vi "Playground.vi"() -> ()   [LabVIEW 2020]
uses:
  Maui 2.0/Maui 2.0.lvclass
  C:/Program Files (x86)/National Instruments/LabVIEW 2020/vi.lib/JKI/JKI SMO/SMO/SMO.lvclass
  <vilib>/JKI/JKI SMO/SMO/SMO.lvclass
panel:
  in  "Stop":bool
  in  "Ring 2":u16(ring) items=["Maui 2.0", "None"]
  in  "Ring":u16(ring) items=["Maui 2.0", "None"]
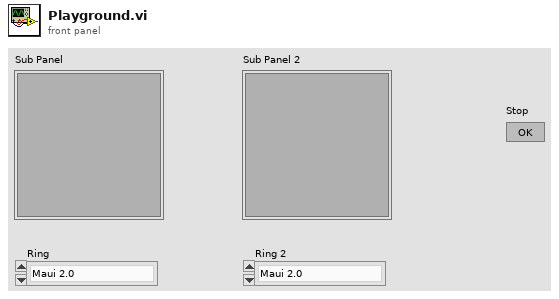
[diagram p1: front panel]
types:
  T1 = cluster{"Ring":refnum<vi>, "Sub Panel":refnum<vi>}
  T2 = cluster{"Ring 2":refnum<vi>, "Sub Panel 2":refnum<vi>}
  T3 = cluster{"Ring 2":refnum<vi>, "Sub Panel 2":refnum<vi>}[]
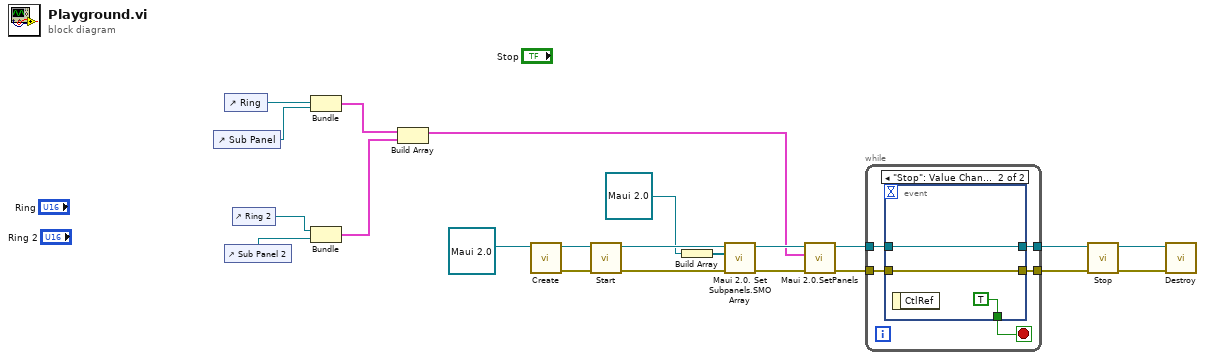
[diagram p0: block diagram]
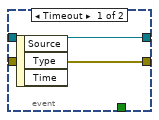
[diagram p2: hidden frame]
diagram:
  n1 = control-ref of="Sub Panel"() -> (w21:refnum<vi>)
  n2 = control-ref of="Ring"() -> (w22:refnum<vi>)
  n3 = control-ref of="Sub Panel 2"() -> (w19:refnum<vi>)
  n4 = control-ref of="Ring 2"() -> (w20:refnum<vi>)
  n5 = Bundle("Ring"=w22, "Sub Panel"=w21) -> (w18:T1)  [unwired: 1 in]
  n6 = Bundle("Ring 2"=w20, "Sub Panel 2"=w19) -> (w17:T2)  [unwired: 1 in]
  n7 = Build Array(w18, w17) -> (w5:T3)
  n8 = call <vilib>:"Create.vi"("SMO"=refnum<class "Maui 2.0.lvclass"> refnum ("Maui 2.0 in")) -> ("error out"=w10:errorcluster, "SMO out"=w15:refnum<class "Maui 2.0.lvclass">)  [unwired: 8 in, 1 out]
  n9 = call <vilib>:"Start.vi"("error in (no error)"=w10, "SMO"=w15) -> ("error out"=w9:errorcluster, "SMO out"=w14:refnum<class "Maui 2.0.lvclass">)  [unwired: 8 in]
  n10 = Build Array(refnum<class "Maui 2.0.lvclass"> refnum ("Maui 2.0 in")) -> (w12:refnum<class "Maui 2.0.lvclass">[])
  n11 = call-dynamic "Maui 2.0. Set Subpanels.SMO Array.vi"("error in (no error)"=w9, "Subpanels in"=w12, "Maui 2.0 in"=w14) -> ("error out"=w6:errorcluster, "Maui 2.0 out"=w7:refnum<class "Maui 2.0.lvclass">)  [unwired: 6 in, 1 out]
  n12 = call "Maui 2.0.SetPanels.vi"("error in (no error)"=w6, "Set Panels"=w5, "Maui 2.0"=w7) -> ("error out"=w3:errorcluster, "Maui 2.0 out"=w4:refnum<class "Maui 2.0.lvclass">)  [unwired: 7 in]
  n13 = while {
    tunnel: w4 -> [w26]
    tunnel: w3 -> [w25]
    tunnel: [w24] -> w1
    tunnel: [w23] -> w2
    stop <- w27 stop-if-true
    n14 = event shown="[1] \"Stop\": Value Change" {
      selector: _ -> [_ _]
      dyn-events: _ -> [_ _]
      timeout: _ -> [_ _]
      tunnel: [_ TRUE] -> w27
      tunnel: w26 -> [w29 w31]
      tunnel: [w29 w31] -> w23
      tunnel: w25 -> [w28 w30]
      tunnel: [w28 w30] -> w24
      event Timeout {
        n15 = event-data() -> ()  [unwired: 1 in, 3 out]
      }
      event "Stop": Value Change {
        n16 = event-data() -> ()  [unwired: 1 in, 1 out]
      }
    }
  }
  n17 = call <vilib>:"Stop.vi"("error in (no error)"=w1, "SMO"=w2) -> ("error out"=w8:errorcluster, "SMO out"=w11:refnum<class "Maui 2.0.lvclass">)  [unwired: 8 in]
  n18 = call <vilib>:"Destroy.vi"("error in (no error)"=w8, "SMO"=w11) -> ()  [unwired: 9 in, 1 out]
